vi "Rotation.vi"(8 "error in (no error)":errorcluster, 9 "Time":dbl, 10 "Direction":dbl) -> (0 "error out":errorcluster, 2 "Done":bool)   [LabVIEW 2019]
uses:
  Timer.vi
  Simulated Robot/Simulation SubVIs/Simulation SubVIs.lvlib
panel:
  out "relative seconds":dbl format="%_19f"
  out "Right 2":dbl
  out "Left 2":dbl
  out "Left":dbl
  out "Right":dbl
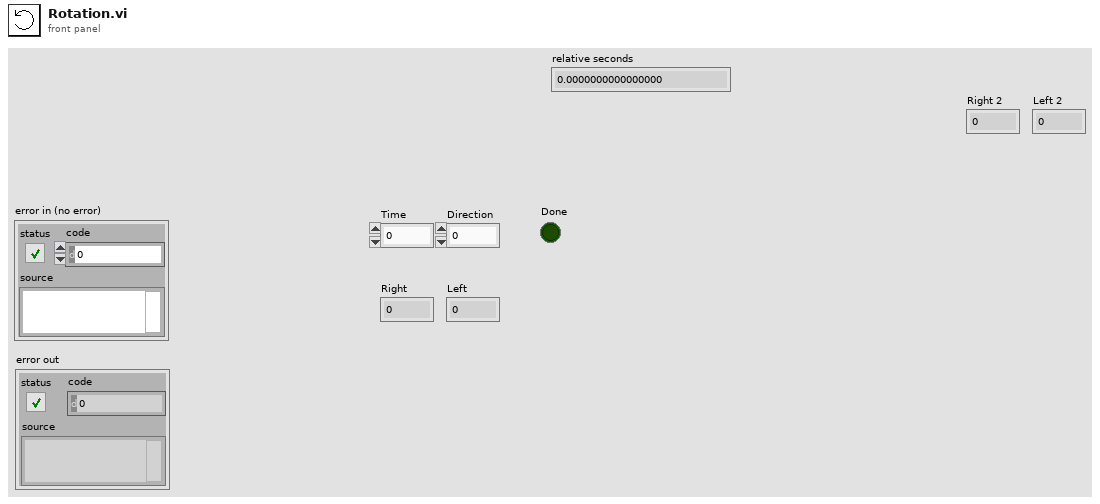
[diagram p1: front panel]
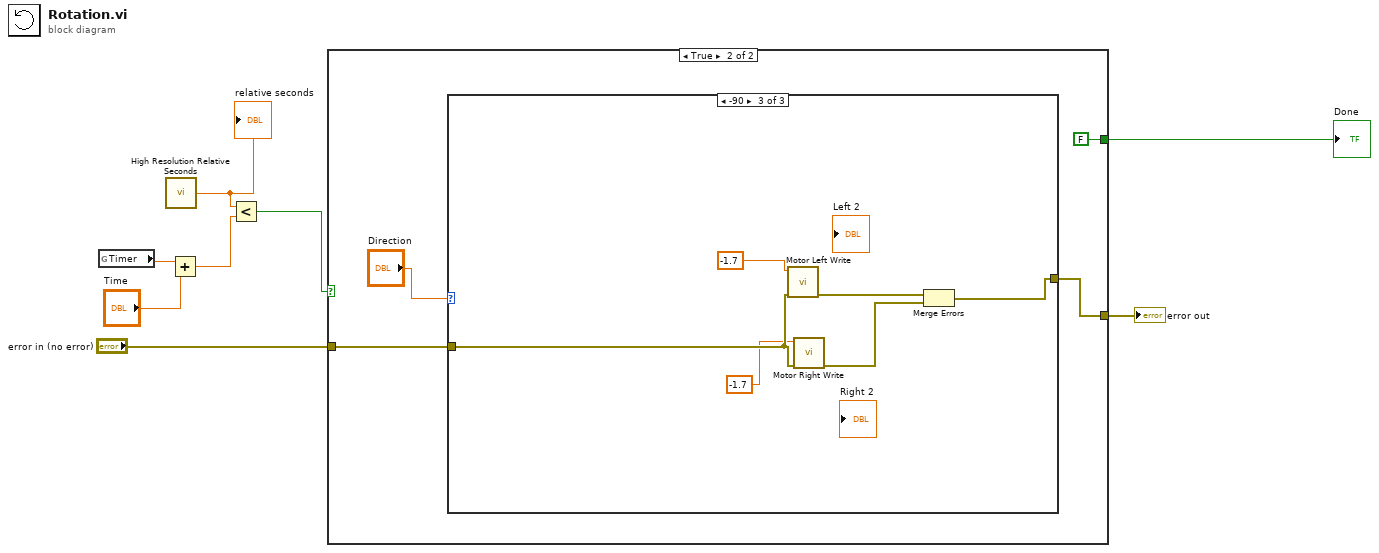
[diagram p0: block diagram]
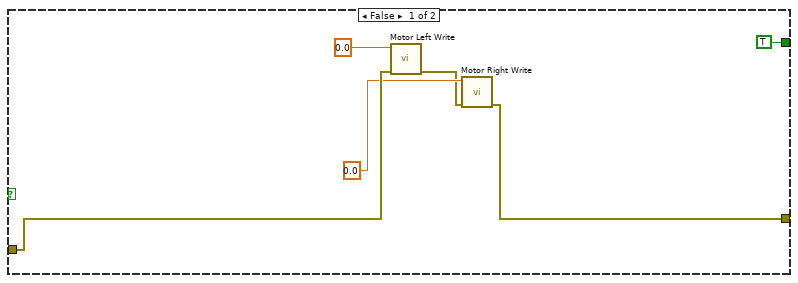
[diagram p2: hidden frame]
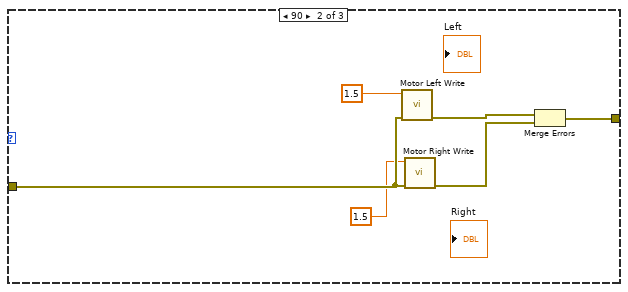
[diagram p4: hidden frame]
diagram:
  n1 = global read "Timer.vi" "Timer"() -> (w3:dbl)
  n2 = call <vilib>:"High Resolution Relative Seconds.vi"() -> ("relative seconds"=w4:dbl)
  "relative seconds" <- w4
  n3 = Add(x=w3, y="Time") -> (x+y=w2:dbl)
  n4 = Less?(x=w4, y=w2) -> (x < y?=w6:bool)
  n5 = case shown="True" w6 {
    tunnel: [w9 w18] -> w8
    tunnel: "error in (no error)" -> [w12 w17]
    tunnel: [TRUE ("Done") FALSE ("Done")] -> w5
    frame False {
      n6 = call "Motor Left Write.vi"("error in (no error)"=w12, "left motor ccw velocity (rad/s)"=0.0) -> ("error out"=w10:errorcluster)  [unwired: 9 in]
      n7 = call "Motor Right Write.vi"("error in (no error)"=w10, "right motor ccw velocity (rad/s)"=0.0) -> ("error out"=w9:errorcluster)  [unwired: 9 in]
    }
    frame True {
      n8 = case shown="-90" "Direction" {
        tunnel: [w19 w23 w29] -> w18
        tunnel: w17 -> [w19 w22 w28]
        frame 0, Default {
        }
        frame 90 {
          n9 = call "Motor Left Write.vi"("error in (no error)"=w22, "left motor ccw velocity (rad/s)"=1.5) -> ("error out"=w24:errorcluster)  [unwired: 9 in]
          n10 = call "Motor Right Write.vi"("error in (no error)"=w22, "right motor ccw velocity (rad/s)"=1.5) -> ("error out"=w25:errorcluster)  [unwired: 9 in]
          n11 = Merge Errors(w24, w25) -> (w23:errorcluster)
        }
        frame -90 {
          n12 = call "Motor Left Write.vi"("error in (no error)"=w28, "left motor ccw velocity (rad/s)"=-1.7) -> ("error out"=w31:errorcluster)  [unwired: 9 in]
          n13 = call "Motor Right Write.vi"("error in (no error)"=w28, "right motor ccw velocity (rad/s)"=-1.7) -> ("error out"=w30:errorcluster)  [unwired: 9 in]
          n14 = Merge Errors(w31, w30) -> (w29:errorcluster)
        }
      }
    }
  }
  "error out" <- w8
  "Done" <- w5
